vi "Peer To Peer Writer - Basic (FPGA).vi"() -> ()   [LabVIEW 2018]
uses:
  <vilib>/Platform/TimedLoop/XDataNode/timing_clust.ctl
  <vilib>/Platform/TimedLoop/XDataNode/nitl_modes.ctl
  <vilib>/Platform/TimedLoop/XDataNode/wakeup.ctl
  <vilib>/rvi/DataTransferAndStorage/FIFO/niFpgaPeerToPeerStreamState.ctl
  <vilib>/rvi/Emulation/niFpgaSctlEmulationGetInTimedLoop.vi
  <vilib>/rvi/Emulation/niFpgaEmulationReportErrorSimple.vi
  <vilib>/rvi/Emulation/niFpgaGetClockAttributes.vi
  <vilib>/rvi/Emulation/niFpgaCriticalErrorInLSC.vi
  <vilib>/rvi/Emulation/niFpgaEmulationIsFPGAContextNoSignature.vi
  <vilib>/rvi/DataTransferAndStorage/Container/Common/niFpgaContainerGetUniqueNameForEmu.vi
  <vilib>/rvi/Memory/Memory_Emulation/niFpgaMemoryEmulationCacheClearOnFirstRun.vi
  <vilib>/rvi/Memory/Memory_Emulation/nirvimemoryEmulationManagerCache_MakeExclusive.vi
  <vilib>/rvi/Memory/Memory_Emulation/niFpgaMemoryEmulationValidateCache.vi
  <vilib>/rvi/Memory/Memory_Emulation/nirvimemoryEmulationManagerCache_InsertValue.vi
  <vilib>/Utility/error.llb/Clear Errors.vi
  <vilib>/rvi/Memory/Memory_Emulation/nirvimemoryEmulationManagerCache_ReleaseExclusive.vi
  <vilib>/rvi/Memory/Memory_Emulation/nirvimemoryEmulationManagerCache_GetValue.vi
  <vilib>/rvi/Memory/Memory_Emulation/nirvimemoryEmulationManagerCache_SetValue.vi
  <vilib>/rvi/Emulation/niFpgaProcessEmulError.vi
  <vilib>/rvi/DataTransferAndStorage/Container/Common/niFpgaContainerSetEmuInfo.vi
  <vilib>/rvi/eio/common/nirviEmuReportErrorAndStop.vi
  <vilib>/Platform/TimedLoop/XDataNode/XDataNode.xnode
  <vilib>/rvi/DataTransferAndStorage/Container/XNode/niFpgaContainer.xnode
  <vilib>/rvi/DataTransferAndStorage/Register/Emulation/niFpgaRegisterEmulation.vi
  <vilib>/rvi/FIFO/Fifo_Resource/nirvififoEmulationP2P.vi
  <vilib>/rvi/LocalResourceManager/LocalResourceManager.xnode
  <vilib>/Platform/TimedLoop/XDataNode/XDNodeRunTimeDep.lvlib
panel:
  out "Samples Sent":u64
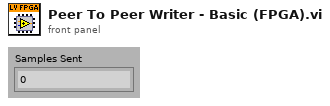
[diagram p1: front panel]
types:
  T1 = typedef "XDNodeRunTimeDep.lvlib/timing_clust.ctl" = cluster{"Expected End [f-1]":u64, "Actual End [f-1]":u64, "Finished Late? [f-1]":bool, "Expected End [i-1]":u64, "Actual End [i-1]":u64, "Finished Late? [i-1]":bool, "Expected Start [i]":u64, "Actual Start [i]":u64, "Expected Start [f]":u64, "Actual Start [f]":u64, "Source Name":string, "Structure Name":string, "Period":i64, "Deadline":i64, "Offset":i64, "Start":i64, "Priority":i32, "Timeout":i32, "Mode":T2, "Wakeup Reason":T3, "Error":errorcluster, "Source Type":string, "Secondary Source Type":string, "Global End Time":u64, "Global Start Time":u64, "Frame Duration":u64, "Iteration Duration":u64, "Assigned CPU":i32, "I/O Scan Engine Mode":u32}
  T2 = typedef "XDNodeRunTimeDep.lvlib/nitl_modes.ctl" = enum32{"No Change", "Process missed periods, maintain original phase", "Discard missed periods, maintain original phase", "Process missed periods, ignore original phase", "Discard missed periods, ignore original phase"}
  T3 = typedef "XDNodeRunTimeDep.lvlib/wakeup.ctl" = enum32{"Normal", "Aborted", "Asynchronous wakeup", "Timing source error", "Timed loop error", "Timeout"}
  T4 = typedef "niFpgaPeerToPeerStreamState.ctl" = enum16{"Unlinked", "Disabled", "Enabled", "Flushing"}
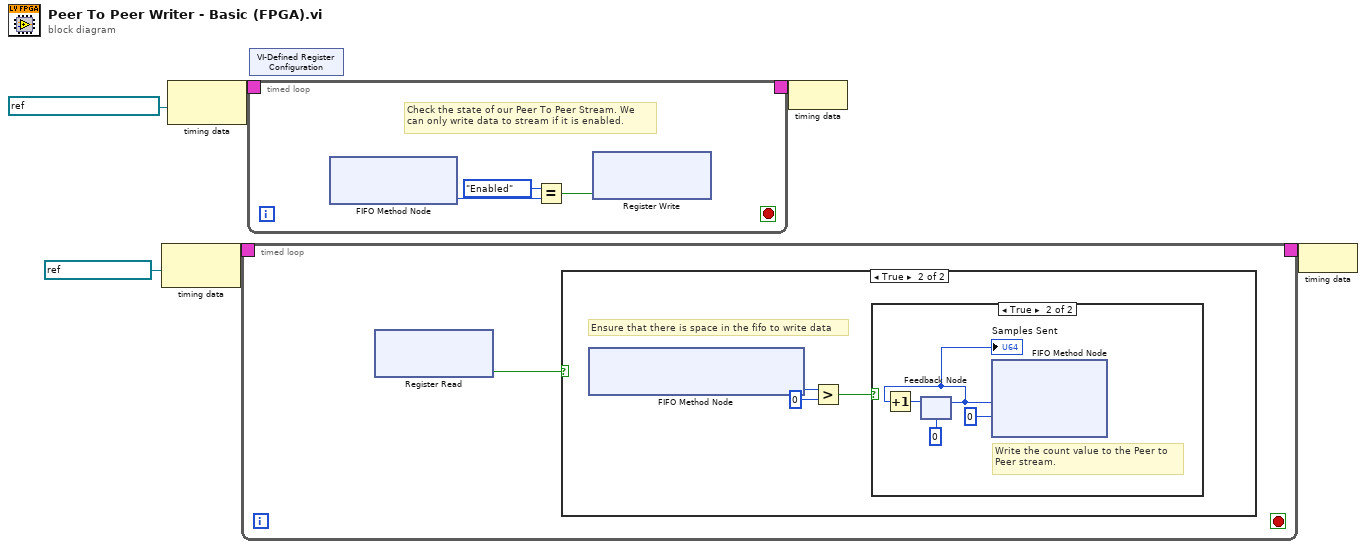
[diagram p0: block diagram]
diagram:
  n1 = node-c288(refnum<k21> "100 MHz Clock" ("Source Name")) -> (w6:T1)
  n2 = node-c288(refnum<k21> "40 MHz Onboard Clock" ("Source Name")) -> (w3:T1)
  n3 = timed-loop {
    timing: w6 -> [_]
    timing-out: [_] -> w5
    stop <- _ stop-if-true
    n4 = xnode ("Register Read")() -> ("Data"=w7:bool)  [unwired: 1 in, 1 out]
    n5 = case shown="True" w7 {
      frame False {
      }
      frame True {
        # "Ensure that there is space in the fifo to write data"
        n6 = xnode ("FIFO Method Node")() -> ("Number of Elements to Write"=w10:u32)  [unwired: 1 in, 1 out]
        n7 = Greater?(x=w10, y=u32 0) -> (0:w8:bool)
        n8 = case shown="True" w8 {
          frame False {
          }
          frame True {
            # "Write the count value to the Peer to\nPeer stream."
            n9 = feedback #1(u64 0 ("Element")) -> (w11:u64)
            "Samples Sent" <- w11
            n10 = Increment(x=w11) -> (x+1=w12:u64)
            n11 = feedback-in #1(w12) -> ()
            n12 = xnode ("FIFO Method Node")("Element"=w11, "Timeout"=0) -> ()  [unwired: 1 in, 2 out]
          }
        }
      }
    }
  }
  n13 = timed-loop {
    timing: w3 -> [_]
    timing-out: [_] -> w2
    stop <- _ stop-if-true
    # "Check the state of our Peer To Peer Stream. We\ncan only write data to stream if it is enabled."
    n14 = xnode ("FIFO Method Node")() -> ("State"=w18:T4)  [unwired: 1 in, 1 out]
    n15 = Equal?(x=niFpgaPeerToPeerStreamState."Enabled", y=w18) -> (x = y?=w17:bool)
    n16 = xnode ("Register Write")("Data"=w17) -> ()  [unwired: 1 in, 1 out]
  }
  n17 = xnode ("VI-Defined Register Configuration")() -> ()  [unwired: 1 out]
  n18 = node-c288(w2) -> ()
  n19 = node-c288(w5) -> ()
